vi "Add Hardware.vi"(8 "error in (no error)":errorcluster, 10 "Hardware.lvclass":refnum<class "Hardware.lvclass">, 11 "Controller in":refnum<class "Controller.lvclass">) -> (0 "error out":errorcluster, 3 "Controller out":refnum<class "Controller.lvclass">)   [LabVIEW 2016, in "Controller Actor.lvlib" / "Controller.lvclass"]
uses:
  <userlib>/Common Components/Controller/Controller.lvclass
  C:/Program Files (x86)/National Instruments/LabVIEW 2016/vi.lib/ActorFramework/Actor/Actor.lvclass
  <userlib>/Common Components/Hardware/Abstract Hardware/Hardware.lvclass
  <vilib>/ActorFramework/Actor/Actor.lvclass/Actor.ctl
  <vilib>/ActorFramework/Message Enqueuer/Message Enqueuer.lvclass/Message Enqueuer.ctl
  <vilib>/ActorFramework/Message Enqueuer/Init from Existing Queue.vi
  <vilib>/ActorFramework/Message Enqueuer/Message Enqueuer.lvclass
  <userlib>/Common Components/Controller/Messages/Log Status/Log Status.lvclass
  <vilib>/ActorFramework/Actor/Actor.lvclass
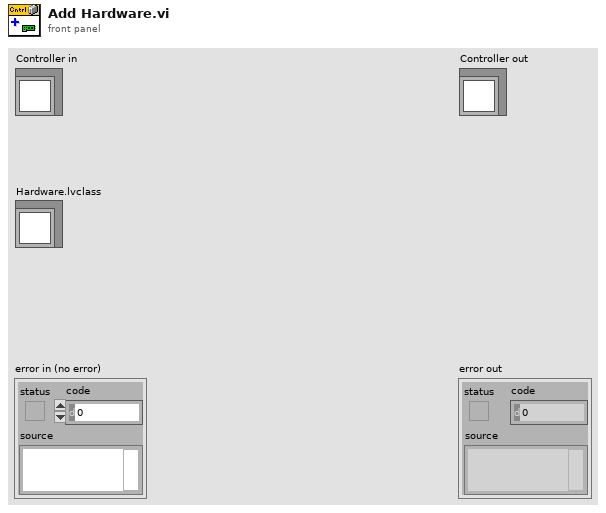
[diagram p1: front panel]
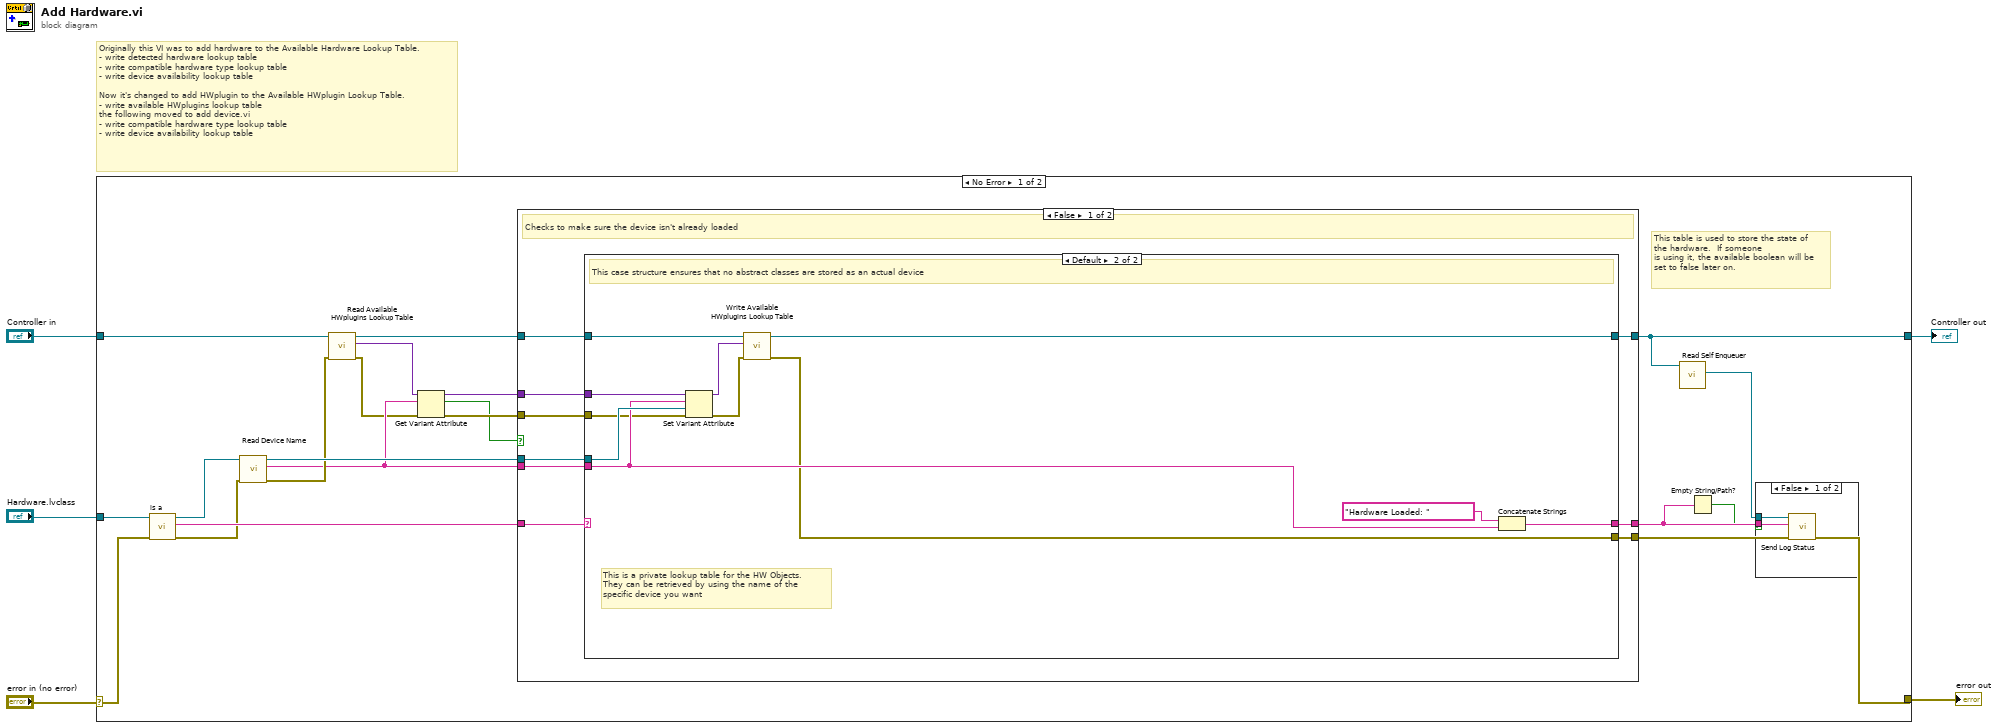
[diagram p0: block diagram]
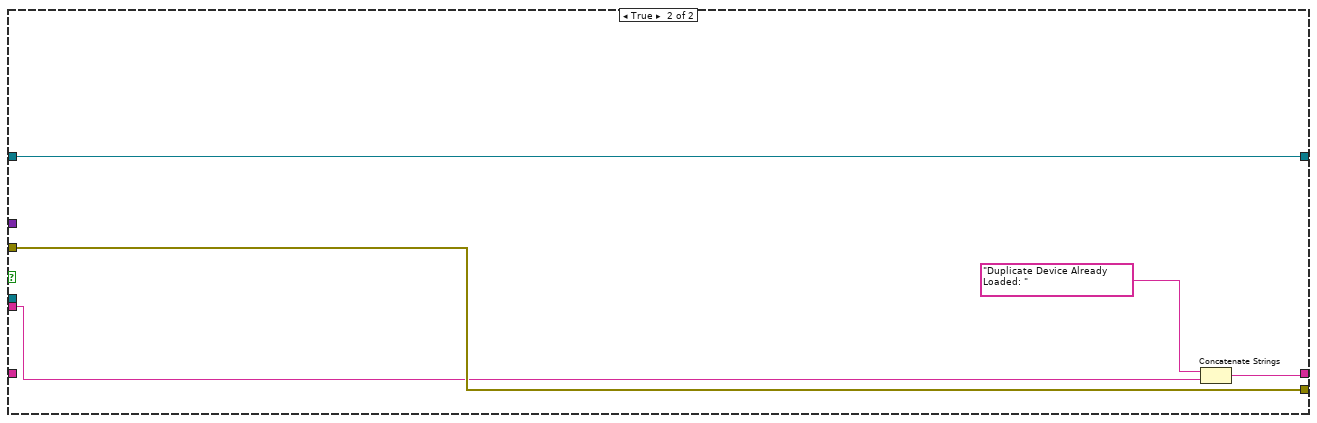
[diagram p4: hidden frame]
diagram:
  # "Originally this VI was to add hardware to the Available Hardware Lookup Table.\n- write detected hardware lookup table\n- write compatible hardware type lookup table\n- write device availability lookup table\n\nNow it's changed to add HWplugin to the Available HWplugin Lookup Table.\n- write available HWplugins lookup table\nthe following moved to add device.vi\n- write compatible hardware type lookup table\n- write device availability lookup table"
  n1 = case shown="No Error" "error in (no error)" {
    selector: "error in (no error)" -> [w24 w56]
    tunnel: [w23 w56] -> w4
    tunnel: [w9 w55] -> w2
    tunnel: "Controller in" -> [w18 w55]
    tunnel: "Hardware.lvclass" -> [w21 _]
    frame No Error {
      # "This table is used to store the state of the hardware.  If someone\nis using it, the available boolean will be set to false later on."
      n2 = call-dynamic "is a.vi"("error in (no error)"=w24, "Hardware in"=w21) -> ("error out"=w19:errorcluster, "is a"=w25:string, "Hardware out"=w20:refnum<class "Hardware.lvclass">)  [unwired: 7 in]
      n3 = call <userlib>:"Read Device Name.vi"("error in (no error)"=w19, "Analog in"=w20) -> ("error out"=w16:errorcluster, "Device Name"=w13:string, "Analog out"=w22:refnum<class "Hardware.lvclass">)  [unwired: 7 in]
      n4 = call <userlib>:"Read Available HWplugins Lookup Table.vi"("error in (no error)"=w16, "Controller in"=w18) -> ("error out"=w12:errorcluster, "Available HWplugins Lookup Table"=w15:variant, "Controller out"=w17:refnum<class "Controller.lvclass">)  [unwired: 7 in]
      n5 = Get Variant Attribute(Variant=w15, name=w13, error in=w12) -> (duplicate Variant=w14:variant, found=w8:bool, error out=w11:errorcluster)  [unwired: 1 in, 1 out]
      n6 = case shown="False" w8 {
        tunnel: w25 -> [w36 _]
        tunnel: [w35 w53] -> w23
        tunnel: w22 -> [w34 _]
        tunnel: w17 -> [w33 w54]
        tunnel: w14 -> [w32 _]
        tunnel: w13 -> [w31 w50]
        tunnel: w11 -> [w30 w53]
        tunnel: [w29 w54] -> w9
        tunnel: [w28 w51] -> w7
        frame False {
          # "Checks to make sure the device isn't already loaded"
          n7 = case shown="Default" w36 {
            tunnel: w33 -> [w38 w44]
            tunnel: [w38 w40] -> w29
            tunnel: [w37 w39] -> w35
            tunnel: w34 -> [_ w46]
            tunnel: w31 -> [_ w45]
            tunnel: w32 -> [_ w43]
            tunnel: w30 -> [w37 w42]
            tunnel: [_ w41] -> w28
            frame "Abstract Class" {
            }
            frame Default {
              # "This is a private lookup table for the HW Objects.  \nThey can be retrieved by using the name of the\nspecific device you want"
              # "This case structure ensures that no abstract classes are stored as an actual device"
              n8 = Set Variant Attribute(Variant=w43, name=w45, value=w46, error in=w42) -> (Variant out=w49:variant, error out=w48:errorcluster)  [unwired: 1 out]
              n9 = call <userlib>:"Write Available HWplugins Lookup Table.vi"("error in (no error)"=w48, "Available HWplugins Lookup Table"=w49, "Controller in"=w44) -> ("error out"=w39:errorcluster, "Controller out"=w40:refnum<class "Controller.lvclass">)  [unwired: 7 in]
              n10 = Concatenate Strings("Hardware Loaded: " ("string"), w45) -> (w41:string)
            }
          }
        }
        frame True {
          n11 = Concatenate Strings("Duplicate Device Already Loaded: " ("string"), w50) -> (w51:string)
        }
      }
      n12 = call <vilib>:"Read Self Enqueuer.vi"("Actor"=w9) -> ("Self Enqueuer"=w10:refnum<class "Message Enqueuer.lvclass">)  [unwired: 10 in]
      n13 = Empty String/Path?(string/path=w7) -> (empty?=w6:bool)
      n14 = case shown="False" w6 {
        tunnel: w10 -> [w27 _]
        tunnel: w7 -> [w26 _]
        frame False {
          n15 = call <userlib>:"Send Log Status.vi"("String"=w26, "Message Enqueuer in"=w27) -> ()  [unwired: 8 in, 2 out]
        }
        frame True {
        }
      }
    }
    frame Error {
    }
  }
  "error out" <- w4
  "Controller out" <- w2
